vi "Get Local and ECAT Config.vi"(6 "fpga wait (s)":u16, 8 "error in (no error)":errorcluster, 11 "Device Reference in":T2 format="%.0x") -> (0 "error out":errorcluster, 1 "ECAT Masters":T1[](array[typedef]) {"DS402 Drive ECAT Slaves"."I/O Output Vars"."VS ref" format="%.0x"; "DS402 Drive ECAT Slaves"."I/O Input Vars"."VS ref" format="%.0x"; "DS402 Drive ECAT Slaves"."VS ref" format="%.0x"; "REM IO ECAT Slaves"."I/O Output Vars"."VS ref" format="%.0x"; "REM IO ECAT Slaves"."I/O Imput Vars"."VS ref" format="%.0x"; "REM IO ECAT Slaves"."VS ref" format="%.0x"; "Generic EtherCAT Slaves"."I/O Output Vars"."VS ref" format="%.0x"; "Generic EtherCAT Slaves"."I/O Imput Vars"."VS ref" format="%.0x"; "Generic EtherCAT Slaves"."VS ref" format="%.0x"; "VS ref" format="%.0x"; "EtherCAT Slaves"."FPGA"."VS ref" format="%.0x"; "EtherCAT Slaves"."RSI Modules"."VS ref" format="%.0x"; "EtherCAT Slaves"."VS ref" format="%.0x"}, 2 "Local Chassis":T30[](array[typedef]) {"FPGA"."UDVs"."To FPGA"."VS ref" format="%.0x"; "FPGA"."UDVs"."From FPGA"."VS ref" format="%.0x"; "FPGA"."VS ref" format="%.0x"; "FPGA"."Output Data"."BD Refs"."Data Reference" format="%.0x"; "FPGA"."Input Data"."BD Refs"."Data Reference" format="%.0x"; "RSI Modules"."Module Config Data"."Config Block Data Refs"."Data Reference" format="%.0x"; "RSI Modules"."CDOutput Data"."BD Refs"."Data Reference" format="%.0x"; "RSI Modules"."CDInput Data"."BD Refs"."Data Reference" format="%.0x"; "RSI Modules"."VS ref" format="%.0x"; "VS ref" format="%.0x"}, 3 "Device Reference out":T2 format="%.0x")   [LabVIEW 2016, in "Scan Engine Custom Device.lvlib"]
uses:
  Scan Engine Custom Device.lvlib
  <vilib>/NI Veristand/Custom Device API/Custom Device Item Ref.ctl
  Type Defs/Local Chassis Data.ctl
  Type Defs/RSI Module Data.ctl
  Type Defs/Open Module IOVs.ctl
  Modules.lvlibp/RSI Module/RSI Module.lvclass
  Modules.lvlibp/RSI Module/Module Models.ctl
  Modules.lvlibp/RSI Module/Channel Type.ctl
  Type Defs/Input Data.ctl
  <vilib>/NI Veristand/Custom Device API/Block Data Reference.ctl
  <vilib>/NI Veristand/Custom Device API/Data Reference.ctl
  Type Defs/Output Data.ctl
  Type Defs/Module Config Data.ctl
  Type Defs/Mixed IO.ctl
  Type Defs/FPGA Data.ctl
  Type Defs/UDV Data.ctl
  Type Defs/UDV Data Type.ctl
  Type Defs/FXP Config.ctl
  Type Defs/Mod Size Indexes.ctl
  Type Defs/EtherCAT Master Data.ctl
  Type Defs/EtherCAT Slave Data.ctl
  Type Defs/Generic ECAT Slave RT-Data-Array.ctl
  Type Defs/Generic ECAT Slave Data Cluster.ctl
  Type Defs/Generic ECAT Slave IOV Cluster.ctl
  Type Defs/REM IO ECAT Slave RT-Data-Array.ctl
  Type Defs/REM IO ECAT Slave Data Cluster.ctl
  Type Defs/REM IO ECAT Slave IOV Cluster.ctl
  Type Defs/DS402 Drive ECAT Slave RT-Data-Array.ctl
  Type Defs/DS402 Drive ECAT Slave Data Cluster.ctl
  Type Defs/DS402 Drive ECAT Slave IOV Cluster.ctl
  Type Defs/DS402 Drive ECAT Slave Action IOV Cluster.ctl
  DS402 StateMachine/Library/controls/state.ctl
  <vilib>/NI Veristand/Custom Device API/Custom Device API.lvlib
  DS402 StateMachine/Library/DS402.lvlib
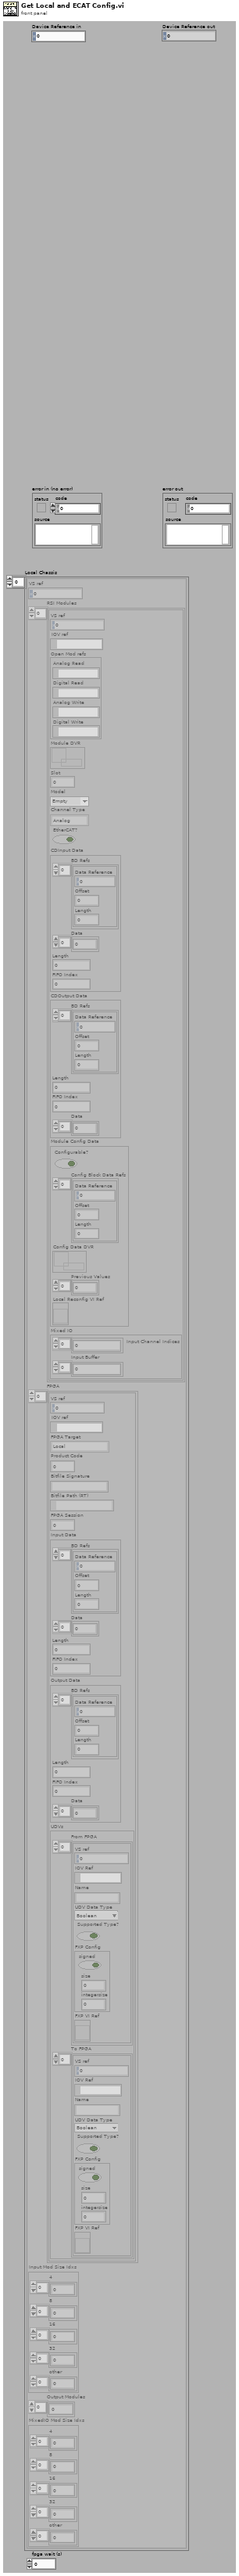
[diagram p1: front panel]
types:
  T1 = typedef "Scan Engine Custom Device.lvlib/EtherCAT Master Data.ctl" = cluster{"VS ref":T2, "IOV ref":refnum<k21>, "Master ID":u32, "Cyclic Data Bandwidth":u32, "EtherCAT Slaves":T3[], "Generic EtherCAT Slaves":T19, "REM IO ECAT Slaves":T22, "DS402 Drive ECAT Slaves":T25}
  T2 = typedef "Custom Device API.lvlib/Custom Device Item Ref.ctl" = u64
  T3 = typedef "Scan Engine Custom Device.lvlib/EtherCAT Slave Data.ctl" = cluster{"VS ref":T2, "IOV ref":refnum<k21>, "Position Address":u16, "RSI Modules":T4[], "FPGA":T14[], "Input Mod Size Idxs":T18, "Output Modules":i32[], "MixedIO Mod Size Idxs":T18}
  T4 = typedef "Scan Engine Custom Device.lvlib/RSI Module Data.ctl" = cluster{"VS ref":T2, "IOV ref":refnum<k21>, "Open Mod refs":T5, "Module DVR":refnum<data-value>, "Slot":u32, "Model":T6, "Channel Type":T7, "EtherCAT?":bool, "CDInput Data":T8, "CDOutput Data":T11, "Module Config Data":T12, "Mixed IO":T13}
  T5 = typedef "Scan Engine Custom Device.lvlib/Open Module IOVs.ctl" = cluster{"Analog Read":refnum<k21>, "Digital Read":refnum<k21>, "Analog Write":refnum<k21>, "Digital Write":refnum<k21>}
  T6 = typedef "Modules.lvlibp/RSI Module.lvclass/Module Models.ctl" = enum16{"Empty", "NI 9201", "NI 9203", "NI 9205", "NI 9206", "NI 9207", "NI 9208", "NI 9211", "NI 9212", "NI 9213", "NI 9214", "NI 9215", "NI 9217", "NI 9219", "NI 9220", "NI 9221", "NI 9222", "NI 9223", "NI 9225", "NI 9227", "NI 9229", "NI 9233", "NI 9234", "NI 9235", "NI 9236", "NI 9237", "NI 9239", "NI 9242", "NI 9244", "NI 9263", "NI 9264", "NI 9265", "NI 9269", "NI 9375", "NI 9401", "NI 9402", "NI 9403", "NI 9411", "NI 9421", "NI 9422", "NI 9423", "NI 9425", "NI 9426", "NI 9435", "NI 9437", "NI 9472", "NI 9474", "NI 9475", "NI 9476", "NI 9477", "NI 9478", "NI 9481", "NI 9482", "NI 9485"}
  T7 = typedef "Modules.lvlibp/RSI Module.lvclass/Channel Type.ctl" = enum16{"Analog", "Digital"}
  T8 = typedef "Scan Engine Custom Device.lvlib/Input Data.ctl" = cluster{"BD Refs":T9[], "Data":dbl[], "Length":i32, "FIFO Index":i32}
  T9 = typedef "Custom Device API.lvlib/Block Data Reference.ctl" = cluster{"Data Reference":T10, "Offset":u64, "Length":u64}
  T10 = typedef "Custom Device API.lvlib/Data Reference.ctl" = i32
  T11 = typedef "Scan Engine Custom Device.lvlib/Output Data.ctl" = cluster{"BD Refs":T9[], "Length":i32, "FIFO Index":i32, "Data":dbl[]}
  T12 = typedef "Scan Engine Custom Device.lvlib/Module Config Data.ctl" = cluster{"Configurable?":bool, "Config Block Data Refs":T9[], "Config Data DVR":refnum<data-value>, "Previous Values":dbl[], "Local Reconfig VI Ref":refnum<vi>}
  T13 = typedef "Scan Engine Custom Device.lvlib/Mixed IO.ctl" = cluster{"Input Channel Indices":i32[], "Input Buffer":dbl[]}
  T14 = typedef "Scan Engine Custom Device.lvlib/FPGA Data.ctl" = cluster{"VS ref":T2, "IOV ref":refnum<k21>, "FPGA Target":enum16{"Local", "EtherCAT"}, "Product Code":u32, "Bitfile Signature":string, "Bitfile Path (RT)":path, "FPGA Session":u32, "Input Data":T8, "Output Data":T11, "UDVs":cluster{"From FPGA":T15[], "To FPGA":T15[]}}
  T15 = typedef "Scan Engine Custom Device.lvlib/UDV Data.ctl" = cluster{"VS ref":T2, "IOV Ref":refnum<k21>, "Name":string, "UDV Data Type":T16, "Supported Type?":bool, "FXP Config":T17, "FXP VI Ref":refnum<vi>}
  T16 = typedef "Scan Engine Custom Device.lvlib/UDV Data Type.ctl" = enum16{"Boolean", "Fixed Point", "Int8", "Int16", "Int32", "Int64", "U32 Bit Field", "UInt8", "UInt16", "UInt32", "UInt64", "Other"}
  T17 = typedef "Scan Engine Custom Device.lvlib/FXP Config.ctl" = cluster{"signed":bool, "size":u32, "integersize":i32}
  T18 = typedef "Scan Engine Custom Device.lvlib/Mod Size Indexes.ctl" = cluster{"4":i32[], "8":i32[], "16":i32[], "32":i32[], "other":i32[]}
  T19 = typedef "Scan Engine Custom Device.lvlib/Generic ECAT Slave RT-Data-Array.ctl" = T20[]
  T20 = typedef "Scan Engine Custom Device.lvlib/Generic ECAT Slave Data Cluster.ctl" = cluster{"VS ref":T2, "IOV ref":refnum<k21>, "Position Address":u16, "I/O Imput Vars ":T21[], "I/O Output Vars":T21[], "I/O Input Data":T8, "I/O Output Data":T11}
  T21 = typedef "Scan Engine Custom Device.lvlib/Generic ECAT Slave IOV Cluster.ctl" = cluster{"VS ref":T2, "IOV Ref":refnum<k21>, "Name":string, "UDV Data Type":T16}
  T22 = typedef "Scan Engine Custom Device.lvlib/REM IO ECAT Slave RT-Data-Array.ctl" = T23[]
  T23 = typedef "Scan Engine Custom Device.lvlib/REM IO ECAT Slave Data Cluster.ctl" = cluster{"VS ref":T2, "IOV ref":refnum<k21>, "Position Address":u16, "I/O Imput Vars ":T24[], "I/O Output Vars":T24[], "I/O Input Data":T8, "I/O Output Data":T11}
  T24 = typedef "Scan Engine Custom Device.lvlib/REM IO ECAT Slave IOV Cluster.ctl" = cluster{"VS ref":T2, "IOV Ref":refnum<k21>, "Name":string, "UDV Data Type":T16, "Scaling Factor":dbl}
  T25 = typedef "DS402 Drive ECAT Slave RT-Data-Array.ctl" = T26[]
  T26 = typedef "Scan Engine Custom Device.lvlib/DS402 Drive ECAT Slave Data Cluster.ctl" = cluster{"VS ref":T2, "IOV ref":refnum<k21>, "Position Address":u16, "I/O Input Vars ":T27[], "I/O Output Vars":T27[], "I/O Input Data":T8, "I/O Output Data":T11, "DS402 IOV":T28}
  T27 = typedef "Scan Engine Custom Device.lvlib/DS402 Drive ECAT Slave IOV Cluster.ctl" = cluster{"VS ref":T2, "IOV Ref":refnum<k21>, "Name":string, "UDV Data Type":T16, "Scaling Factor":dbl, "IOV":bool, "VS data Index":i32}
  T28 = typedef "Scan Engine Custom Device.lvlib/DS402 Drive ECAT Slave Action IOV Cluster.ctl" = cluster{"Control Word":refnum<k21>, "Status Word":refnum<k21>, "Input Offset":i32, "Output Offset":i32, "State":T29}
  T29 = typedef "Scan Engine Custom Device.lvlib/DS402.lvlib/state.ctl" = enum16{"Init", "Not Ready to Switch On", "Read Status Word", "Switch on disabled", "Ready to switch on", "Switched on", "Operation enabled", "Fault", "Fault reaction active", "Quick stop active", "Shutdown - Bad State", "Shutdown - Error", "Shutdown - Normal", "Shutdown - Fault"}
  T30 = typedef "Scan Engine Custom Device.lvlib/Local Chassis Data.ctl" = cluster{"VS ref":T2, "RSI Modules":T4[], "FPGA":T14[], "Input Mod Size Idxs":T18, "Output Modules":i32[], "MixedIO Mod Size Idxs":T18}
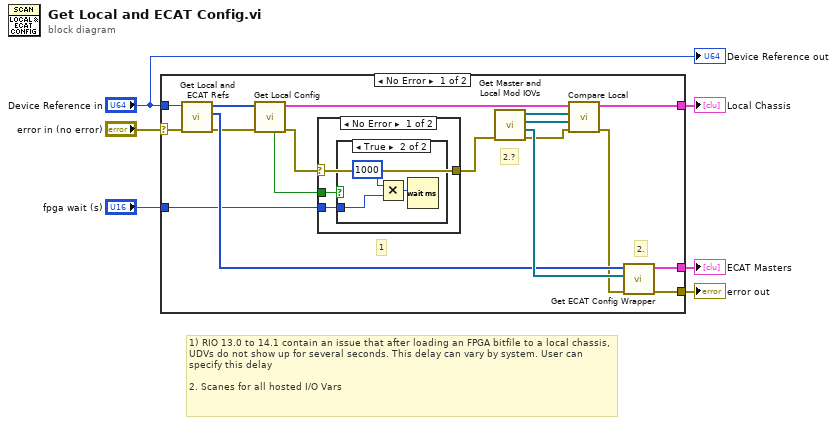
[diagram p0: block diagram]
diagram:
  # "1) RIO 13.0 to 14.1 contain an issue that after loading an FPGA bitfile to a local chassis, UDVs do not show up for several seconds. This delay can vary by system. User can specify this delay\n\n2. Scanes for all hosted I/O Vars"
  n1 = case shown="No Error" "error in (no error)" {
    selector: "error in (no error)" -> [w21 w32]
    tunnel: "Device Reference in" -> [w20 _]
    tunnel: [w23 w32] -> w6
    tunnel: [w16 _] -> w3
    tunnel: [w24 _] -> w2
    tunnel: "fpga wait (s)" -> [w8 _]
    frame No Error {
      # "2."
      # "2.?"
      # "1"
      n2 = call "Get Local and ECAT Refs.vi"("error in (no error)"=w21, "Device Reference in"=w20) -> ("error out"=w12:errorcluster, "ECAT Master Refs"=w19:T2[], "Local Chassis Refs"=w13:T2[])  [unwired: 7 in]
      n3 = call "Get Local Config.vi"("error in (no error)"=w12, "Local Chassis Refs"=w13) -> ("error out"=w10:errorcluster, "Local Chassis"=w11:T30[], "FPGALoaded"=w9:bool)  [unwired: 7 in]
      n4 = case shown="No Error" w10 {
        selector: w10 -> [w26 w31]
        tunnel: w9 -> [w27 _]
        tunnel: [w26 w31] -> w7
        tunnel: w8 -> [w25 _]
        frame No Error {
          n5 = case shown="True" w27 {
            tunnel: w25 -> [_ w30]
            frame False {
            }
            frame True {
              n6 = Multiply(x=u16 1000, y=w30) -> (x*y=w29:u16)
              n7 = Wait (ms)(milliseconds to wait=w29) -> ()  [unwired: 1 out]
            }
          }
        }
        frame Error {
        }
      }
      n8 = call "Get Master and Local Mod IOVs.vi"("error in (no error)"=w7) -> ("error IO"=w18:errorcluster, "All Masters"=w22:refnum<k21>[], "All Local Mods"=w14:refnum<k21>[], "Local UDV Container"=w15:refnum<k21>[])  [unwired: 7 in]
      n9 = call "Compare Local.vi"("error in (no error)"=w18, "All Local Mods"=w14, "Local UDV Container"=w15, "Local Chassis in"=w11) -> ("error out"=w17:errorcluster, "Local Chassis out"=w16:T30[])  [unwired: 6 in]
      n10 = call "Get ECAT Config Wrapper.vi"("error in (no error)"=w17, "All ECAT Masters"=w22, "ECAT Master refs"=w19) -> ("error out"=w23:errorcluster, "ECAT Masters out"=w24:T1[])  [unwired: 7 in]
    }
    frame Error {
    }
  }
  "error out" <- w6
  "Local Chassis" <- w3
  "ECAT Masters" <- w2
  "Device Reference out" <- "Device Reference in"
